vi "GA Loop Condition.vi"(9 "Set Value":bool, 11 "Method":T1) -> (1 "GA Loop Condition Out":bool)   [LabVIEW 2013]
uses:
  GA Loop Condition FGV.ctl
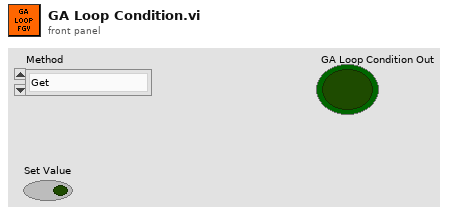
[diagram p1: front panel]
types:
  T1 = typedef "GA Loop Condition FGV.ctl" = enum16{"Get", "Set"}
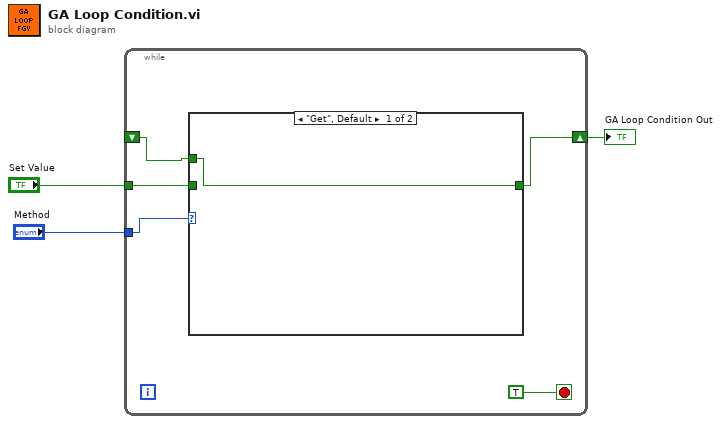
[diagram p0: block diagram]
diagram:
  n1 = while {
    tunnel: "Method" -> [w8]
    shift-right: [w5] -> w1
    shift-left: _ -> [w7]
    tunnel: "Set Value" -> [w6]
    stop <- TRUE stop-if-true
    n2 = case shown="\"Get\", Default" w8 {
      tunnel: w7 -> [w9 _]
      tunnel: w6 -> [_ w10]
      tunnel: [w9 w10] -> w5
      frame "Get", Default {
      }
      frame "Set" {
      }
    }
  }
  "GA Loop Condition Out" <- w1
